vi "getMTInputQty.vi"(9 "Step":string, 11 "rcno":string) -> (0 "error out":errorcluster, 2 "data":i32)   [LabVIEW 2012]
uses:
  <vilib>/addons/database/Auxilliary.llb/DB Tools Cursor Type.ctl
  <vilib>/addons/database/Connection.llb/DB Tools Open Connec (Path).vi
  <vilib>/addons/database/Connection.llb/Conn Execute.vi
  <vilib>/addons/database/Recordset.llb/Rec Fetch Integer Data (R).vi
  <vilib>/addons/database/Recordset.llb/Rec Destroy - Connection.vi
  <vilib>/addons/database/NI_Database_API.lvlib
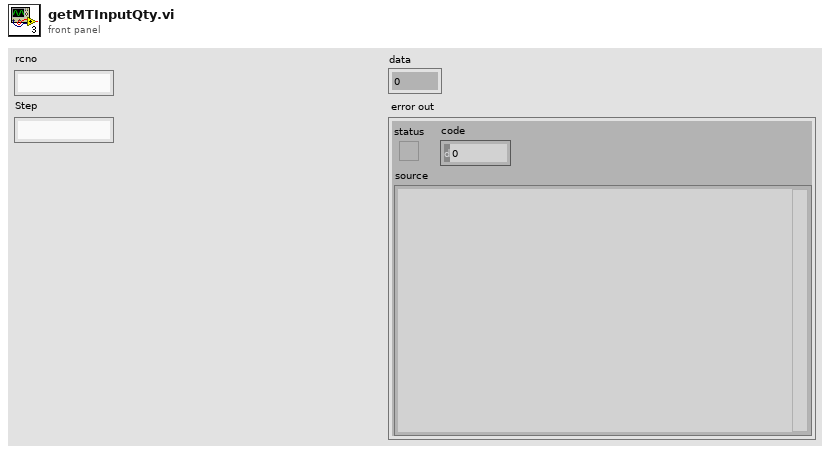
[diagram p1: front panel]
types:
  T1 = typedef "NI_Database_API.lvlib/DB Tools Cursor Type.ctl" = enum16{"forward-only", "keyset", "dynamic", "static"}
  T2 = typedef "NI_Database_API.lvlib/Conn ObjectReference.ctl" = refnum<k1>
  T3 = typedef "NI_Database_API.lvlib/Rec ObjectReference.ctl" = refnum<k1>
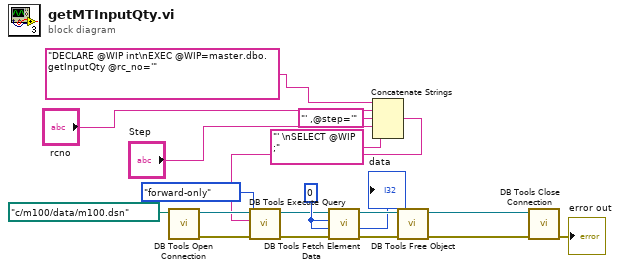
[diagram p0: block diagram]
diagram:
  w6 = 0
  n1 = call-poly <vilib>:"DB Tools Open Connection.vi"("connection information"=path "c:/m100/data/m100.dsn") -> ("error out"=w16:errorcluster, "connection reference"=w19:T2)  [unwired: 7 in]
  n2 = Concatenate Strings("DECLARE @WIP int\nEXEC @WIP=master.dbo.getInputQty @rc_no='" ("SQL query"), "rcno", "' ,@step='" ("string"), "Step", "' \nSELECT @WIP ;" ("string")) -> (w2:string)
  n3 = call-poly <vilib>:"DB Tools Execute Query.vi"("error in (no error)"=w16, "cursor type"=DB_Tools_Cursor_Type."forward-only", "SQL query"=w2, "connection reference"=w19) -> ("error out"=w15:errorcluster, "recordset reference"=w5:T3)  [unwired: 4 in]
  n4 = call-poly <vilib>:"DB Tools Fetch Element Data.vi"("error in (no error)"=w15, "type"=w6, "column index"=w6, "recordset reference"=w5) -> ("error out"=w14:errorcluster, "data"=→"data":i32, "recordset reference out"=w18:T3)  [unwired: 3 in]
  n5 = call-poly <vilib>:"DB Tools Free Object.vi"("error in (no error)"=w14, "recordset reference"=w18) -> ("error out"=w13:errorcluster, "connection reference"=w17:T2)  [unwired: 8 in]
  n6 = call <vilib>:"DB Tools Close Connection.vi"("error in (no error)"=w13, "connection reference"=w17) -> ("error out"=→"error out":errorcluster)  [unwired: 5 in]
